vi "Teleop.vi"(10 "Match Info":T1={"Autonomous Elapsed Seconds"=0.0, "TeleOp Elapsed Seconds"=0.0, "Disabled Elapsed Seconds"=0.0, "Visited Autonomous"=FALSE, "Visited TeleOp"=FALSE, "Visited Disabled"=FALSE, "Autonomous Settings"={"Autonomous Style"=enum."Independent", "VI Refnum"=refnum}}, 11 "Call Context":T2) -> ()   [LabVIEW 2014]
doc: "This VI is called for each TeleOp packet received from the DS where the robot is not disabled. It is often used to read from the joysticks and update I/O or to update setpoints for timed control loops. It should complete and return within 20 milliseconds or it may miss DS packets."
uses:
  <vilib>/Rock Robotics/WPI/DriverStation/WPI_DriverStationDerivedRobotMode.ctl
  <vilib>/Rock Robotics/WPI/DriverStation/WPI_DriverStationMatch Info.ctl
  <vilib>/Rock Robotics/Network Tables/SD Read Boolean.vi
  <vilib>/Rock Robotics/Network Tables/SD Read Number.vi
  <vilib>/Rock Robotics/WPI/Joystick/WPI_JoystickGetSetRefNum.vi
  <vilib>/Rock Robotics/WPI/RobotDrive/WPI_RobotDriveGetSetRefNum.vi
  <vilib>/Rock Robotics/Network Tables/SD Write Numeric Array.vi
  <vilib>/Rock Robotics/Network Tables/SD Write Boolean Array.vi
panel:
  out "Right and Left Drive Motors Indicator":dbl[](array[numeric])
  out "Winch Cim 2 Indicator":dbl
  out "Winch Cim 1 Indicator":dbl
  out "Lower Limit Indicator":bool
  out "Back Ejector Limit Indicator":bool
  out "Left Drive Encoder Indicator":dbl
  out "Right Drive Encoder Indicator":dbl
  out "Front Ejector Limit Indicator":bool
  out "Claw Open Limit Indicator":bool
  out "Claw Closed Limit Indicator":bool
  out "Upper Limit Indicator":bool
  out "Buttons":bool[](array[boolean])
  out "Axes":dbl[](array[numeric])
  out "Sample Slider 0":dbl(slide) scale=0.0..5.0
  out "Sample Boolean 1":bool
  out "Sample Boolean 0":bool
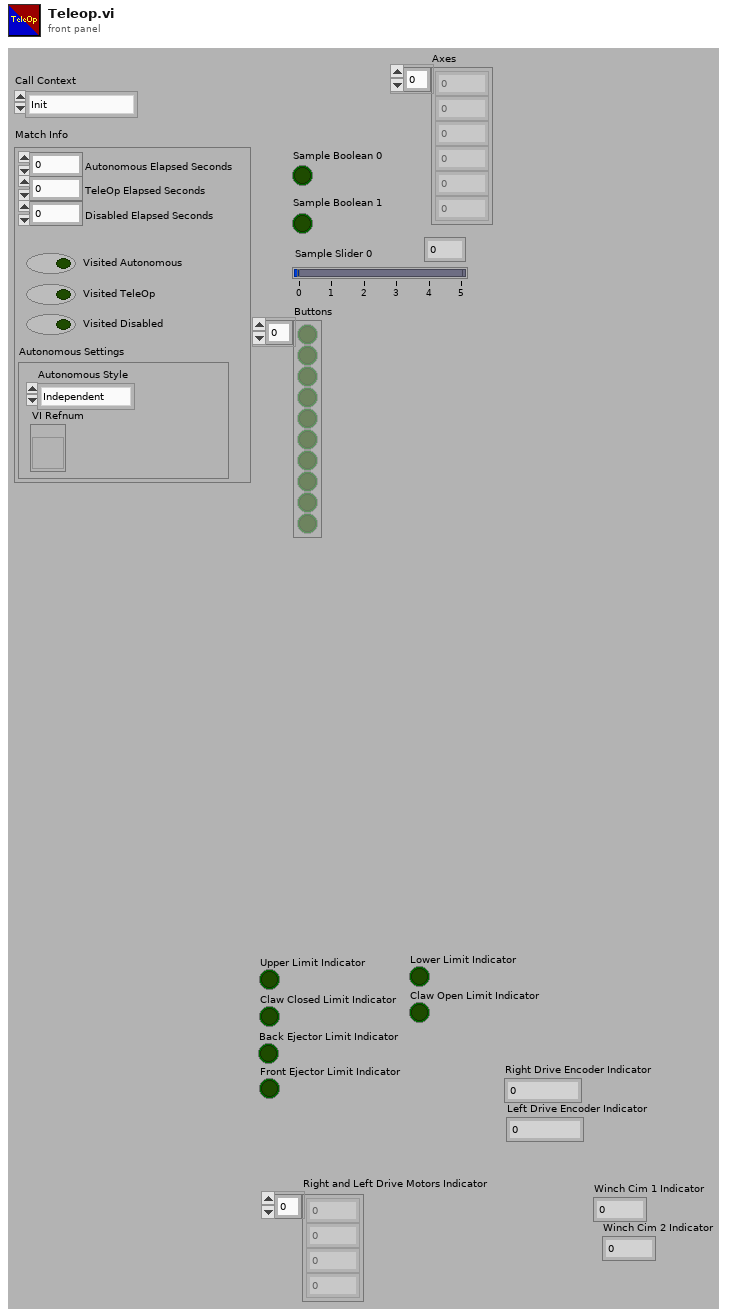
[diagram p1: front panel]
types:
  T1 = typedef "WPI_DriverStationMatch Info.ctl" = cluster{"Autonomous Elapsed Seconds":dbl, "TeleOp Elapsed Seconds":dbl, "Disabled Elapsed Seconds":dbl, "Visited Autonomous":bool, "Visited TeleOp":bool, "Visited Disabled":bool, "Autonomous Settings":cluster{"Autonomous Style":enum16{"Iterative", "Independent"}, "VI Refnum":refnum<vi>}}
  T2 = typedef "WPI_DriverStationDerivedRobotMode.ctl" = enum16{"Init", "Execute", "Stop"}
  T3 = typedef "WPI_RobotDriveDevRef.ctl" = cluster{"DevStatus":errorcluster, "Motors[]":T4[], "Square Inputs":bool, "Max Output":dbl}
  T4 = typedef "WPI_MotorControlDeviceRef.ctl" = cluster{"DeviceStatus":errorcluster, "Type":T5, "PWM":cluster{"Controller":T6, "PWM Channel":T7, "DeadBand":T8}, "CAN":cluster{"Device Number":u8, "Control Mode":T9, "Semaphore":T10, "Max Vout":dbl, "TalonSRX Control Mode":T11}, "Invert":bool, "TransformRef":T12, "InvTransformRef":T12}
  T5 = typedef "WPI_MotorControlType.ctl" = enum16{"PWM", "CAN", "CANTalonSRX"}
  T6 = typedef "FPGA_TypedefDigitalModule.ctl" = enum16{"Controller 1"}
  T7 = typedef "FPGA_DIOPWMChannel.ctl" = enum8{"PWM 0", "PWM 1", "PWM 2", "PWM 3", "PWM 4", "PWM 5", "PWM 6", "PWM 7", "PWM 8", "PWM 9", "PWM MXP 0", "PWM MXP 1", "PWM MXP 2", "PWM MXP 3", "PWM MXP 4", "PWM MXP 5", "PWM MXP 6", "PWM MXP 7", "PWM MXP 8", "PWM MXP 9", "Invalid"}
  T8 = typedef "WPI_PWMDeadband.ctl" = cluster{"Name":string, "maxPositivePwm":i32, "minPositivePwm":i32, "centerPwm":i32, "maxNegativePwm":i32, "minNegativePwm":i32, "angularRange":u16}
  T9 = typedef "WPI_CANJaguar_ControlMode.ctl" = enum8{"Percent VBus", "Current", "Speed", "Position", "Voltage"}
  T10 = typedef "Semaphore RefNum" = refnum<k1>
  T11 = typedef "WPI_CANTalonSRX_APIControlMode.ctl" = enum8{"Percent VBus", "Speed", "Position", "Slave", "Unchanged / Invalid"}
  T12 = typedef "WPI_PWMTransform_ConPane.ctl" = refnum<vi>
  T13 = typedef "WPI_JoystickDevRef.ctl" = cluster{"Device":T14}
  T14 = typedef "WPI_JoystickDeviceEnum.ctl" = enum16{"USB 0", "USB 1", "USB 2", "USB 3", "USB 4", "USB 5"}
  T15 = cluster{"Axes[0]":dbl, "Axes[1]":dbl, "Axes[2]":dbl, "Axes[3]":dbl, "Axes[4]":dbl, "Axes[5]":dbl, "Axes[6]":dbl, "Axes[7]":dbl, "Axes[8]":dbl}
  T16 = cluster{"Buttons[0]":bool, "Buttons[1]":bool, "Buttons[2]":bool, "Buttons[3]":bool, "Buttons[4]":bool, "Buttons[5]":bool, "Buttons[6]":bool, "Buttons[7]":bool, "Buttons[8]":bool}
  T17 = typedef "WPI_DigitalInputDevRef.ctl" = cluster{"DevStatus":errorcluster, "DIO Channel":T18, "Controller":T6}
  T18 = typedef "FPGA_DIOChannel.ctl" = enum8{"DIO 0", "DIO 1", "DIO 2", "DIO 3", "DIO 4", "DIO 5", "DIO 6", "DIO 7", "DIO 8", "DIO 9", "DIO MXP 0", "DIO MXP 1", "DIO MXP 2", "DIO MXP 3", "DIO MXP 4", "DIO MXP 5", "DIO MXP 6", "DIO MXP 7", "DIO MXP 8", "DIO MXP 9", "DIO MXP 10", "DIO MXP 11", "DIO MXP 12", "DIO MXP 13", "DIO MXP 14", "DIO MXP 15", "Invalid"}
  T19 = typedef "WPI_EncoderDevRef.ctl" = cluster{"DevStatus":errorcluster, "EncoderIndex":T20, "CounterIndex":T21, "DistancePerCount":dbl, "Decoding Type":T22}
  T20 = typedef "FPGA_EncoderIdx.ctl" = enum8{"Enc 0", "Enc 1", "Enc 2", "Enc 3", "Enc 4", "Enc 5", "Enc 6", "Enc 7", "Invalid"}
  T21 = typedef "FPGA_CounterCtrSystemIndex.ctl" = enum8{"Ctr 0", "Ctr 1", "Ctr 2", "Ctr 3", "Ctr 4", "Ctr 5", "Ctr 6", "Ctr 7", "Invalid"}
  T22 = typedef "WPI_EncoderType.ctl" = enum16{"1x", "2x", "4x"}
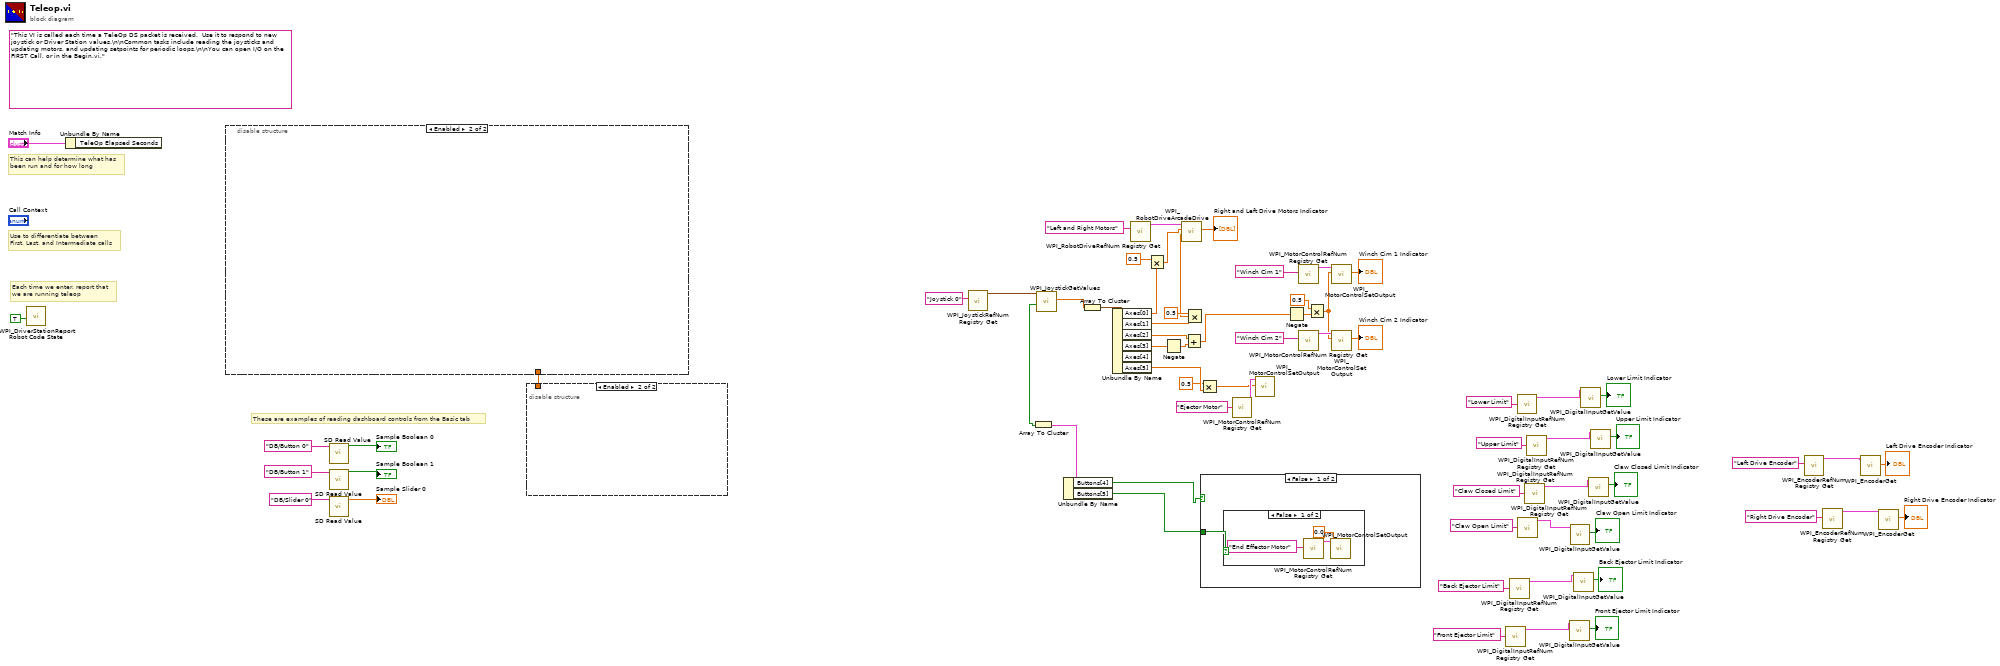
[diagram p0: block diagram]
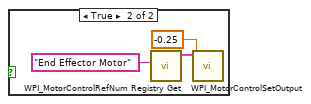
[diagram p2: hidden frame]
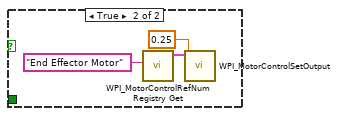
[diagram p3: hidden frame]
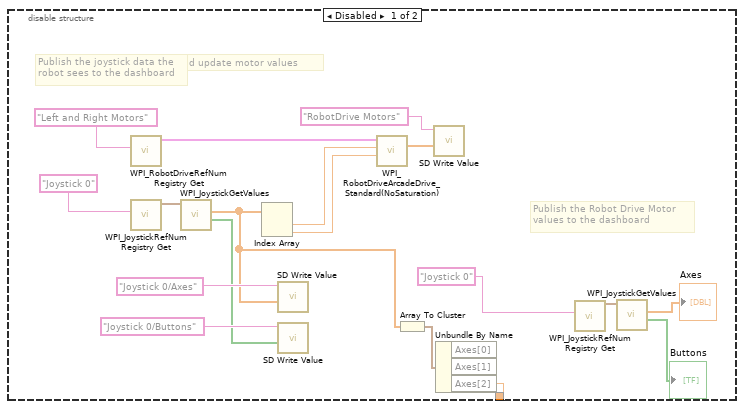
[diagram p4: hidden frame]
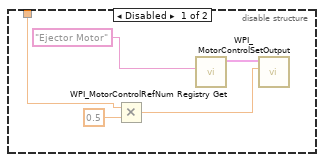
[diagram p5: hidden frame]
diagram:
  (unwired) "This VI is called each time a TeleOp DS packet is received.  Use it to respond to new joystick or Driver Station values.\n\nCommon tasks include reading the joysticks and updating motors, and updating setpoints for periodic loops.\n\nYou can open I/O on the FIRST Call, or in the Begin.vi."
  # "These are examples of reading dashboard controls from the Basic tab"
  # "Each time we enter, report that\nwe are running teleop"
  # "Use to differentiate between\nFirst, Last, and Intermediate calls"
  # "This can help determine what has\nbeen run and for how long"
  n1 = call <vilib>:"WPI_DriverStationReport Robot Code State.vi"("TeleOp"=TRUE ("Autonomous")) -> ()  [unwired: 10 in, 1 out]
  n2 = Unbundle By Name("Match Info") -> ()  [unwired: 1 out]
  n3 = disable-structure shown="Enabled" {
    disable-tunnel: [w69 _] -> w60
    frame Disabled {
      # "Publish the Robot Drive Motor\nvalues to the dashboard"
      # "Publish the joystick data the\nrobot sees to the dashboard"
      # "Read Joystick X and Y values and update motor values"
      n4 = call <vilib>:"WPI_RobotDriveRefNum Registry Get.vi"("refnum name"="Left and Right Motors") -> ("RobotDriveDevRef"=w85:T3)  [unwired: 1 in, 9 out]
      n5 = call <vilib>:"WPI_JoystickRefNum Registry Get.vi"("refnum name"="Joystick 0") -> ("JoystickDevRef"=w82:T13)  [unwired: 1 in, 9 out]
      n6 = call <vilib>:"WPI_JoystickGetValues.vi"("JoystickDevRef"=w82) -> ("Buttons"=w76:bool[], "Axes"=w71:dbl[])  [unwired: 6 in, 3 out]
      n7 = Index Array(array=w71) -> (element #1=w84:dbl, element #2=w80:dbl)  [unwired: 2 in]
      n8 = call-poly <vilib>:"SD Write Value.vi"("Numeric Array"=w71, "Name"="Joystick 0/Axes") -> ()  [unwired: 8 in, 2 out]
      n9 = call-poly <vilib>:"SD Write Value.vi"("Boolean Array"=w76, "Name"="Joystick 0/Buttons") -> ()  [unwired: 8 in, 2 out]
      n10 = call <vilib>:"WPI_RobotDriveArcadeDrive_Standard(NoSaturation).vi"("Y axis value"=w80, "X axis value"=w84, "RobotDriveDevRef"=w85) -> ("Motor Values"=w79:dbl[])  [unwired: 1 in, 7 out]
      n11 = Array To Cluster(array=w71) -> (cluster=w70:T15)
      n12 = call-poly <vilib>:"SD Write Value.vi"("Numeric Array"=w79, "Name"="RobotDrive Motors") -> ()  [unwired: 8 in, 2 out]
      n13 = Unbundle By Name(w70) -> ("Axes[2]"=w69:dbl)  [unwired: 2 out]
      n14 = call <vilib>:"WPI_JoystickRefNum Registry Get.vi"("refnum name"="Joystick 0") -> ("JoystickDevRef"=w74:T13)  [unwired: 9 in, 1 out]
      n15 = call <vilib>:"WPI_JoystickGetValues.vi"("JoystickDevRef"=w74) -> ("Buttons"=→"Buttons":bool[], "Axes"=→"Axes":dbl[])  [unwired: 6 in, 3 out]
    }
    frame Enabled {
    }
  }
  n16 = call-poly <vilib>:"SD Read Value.vi"("Name"="DB/Button 0" ("refnum name")) -> ("Boolean"=→"Sample Boolean 0":bool)  [unwired: 8 in, 2 out]
  n17 = call-poly <vilib>:"SD Read Value.vi"("Name"="DB/Button 1" ("refnum name")) -> ("Boolean"=→"Sample Boolean 1":bool)  [unwired: 8 in, 2 out]
  n18 = call-poly <vilib>:"SD Read Value.vi"("Name"="DB/Slider 0" ("refnum name")) -> ("Numeric"=→"Sample Slider 0":dbl)  [unwired: 8 in, 2 out]
  n19 = disable-structure shown="Enabled" {
    disable-tunnel: w60 -> [w88 _]
    frame Disabled {
      n20 = Multiply(x=w88, y=0.5) -> (x*y=w87:dbl)
      n21 = call <vilib>:"WPI_MotorControlRefNum Registry Get.vi"("refnum name"="Ejector Motor") -> ("MotorControlDevRef"=w90:T4)  [unwired: 9 in, 1 out]
      n22 = call <vilib>:"WPI_MotorControlSetOutput.vi"("Output"=w87, "MotorControlDevRef"=w90) -> ()  [unwired: 7 in, 3 out]
    }
    frame Enabled {
    }
  }
  n23 = call <vilib>:"WPI_JoystickRefNum Registry Get.vi"("refnum name"="Joystick 0") -> ("JoystickDevRef"=w37:T13)  [unwired: 9 in, 1 out]
  n24 = call <vilib>:"WPI_JoystickGetValues.vi"("JoystickDevRef"=w37) -> ("Buttons"=w33:bool[], "Axes"=w35:dbl[])  [unwired: 6 in, 3 out]
  n25 = Array To Cluster(array=w33) -> (cluster=w32:T16)
  n26 = Unbundle By Name(w32) -> ("Buttons[4]"=w5:bool, "Buttons[5]"=w4:bool)
  n27 = Array To Cluster(array=w35) -> (cluster=w34:T15)
  n28 = Unbundle By Name(w34) -> ("Axes[0]"=w7:dbl, "Axes[1]"=w11:dbl, "Axes[2]"=w20:dbl, "Axes[3]"=w21:dbl, "Axes[5]"=w2:dbl)  [unwired: 1 out]
  n29 = call <vilib>:"WPI_RobotDriveRefNum Registry Get.vi"("refnum name"="Left and Right Motors") -> ("RobotDriveDevRef"=w31:T3)  [unwired: 9 in, 1 out]
  n30 = Multiply(x=0.5, y=w7) -> (x*y=w6:dbl)
  n31 = Negate(x=w21) -> (-x=w19:dbl)
  n32 = Add(x=w20, y=w19) -> (x+y=w3:dbl)
  n33 = Multiply(x=0.5, y=w11) -> (x*y=w9:dbl)
  n34 = call-poly <vilib>:"WPI_RobotDriveArcadeDrive.vi"("Y axis value"=w9, "X axis value"=w6, "RobotDriveDevRef"=w31) -> ("Motor Values"=→"Right and Left Drive Motors Indicator":dbl[])  [unwired: 6 in, 2 out]
  n35 = Multiply(x=0.5, y=w2) -> (x*y=w12:dbl)
  n36 = case shown="False" w5 {
    tunnel: w4 -> [w92 _]
    frame False {
      n37 = case shown="False" w92 {
        frame False {
          n38 = call <vilib>:"WPI_MotorControlRefNum Registry Get.vi"("refnum name"="End Effector Motor" ("Name")) -> ("MotorControlDevRef"=w95:T4)  [unwired: 9 in, 1 out]
          n39 = call <vilib>:"WPI_MotorControlSetOutput.vi"("Output"=0.0, "MotorControlDevRef"=w95) -> ()  [unwired: 7 in, 3 out]
        }
        frame True {
          n40 = call <vilib>:"WPI_MotorControlRefNum Registry Get.vi"("refnum name"="End Effector Motor" ("Name")) -> ("MotorControlDevRef"=w98:T4)  [unwired: 9 in, 1 out]
          n41 = call <vilib>:"WPI_MotorControlSetOutput.vi"("Output"=-0.25, "MotorControlDevRef"=w98) -> ()  [unwired: 7 in, 3 out]
        }
      }
    }
    frame True {
      n42 = call <vilib>:"WPI_MotorControlRefNum Registry Get.vi"("refnum name"="End Effector Motor" ("Name")) -> ("MotorControlDevRef"=w101:T4)  [unwired: 9 in, 1 out]
      n43 = call <vilib>:"WPI_MotorControlSetOutput.vi"("Output"=0.25, "MotorControlDevRef"=w101) -> ()  [unwired: 7 in, 3 out]
    }
  }
  n44 = call <vilib>:"WPI_MotorControlRefNum Registry Get.vi"("refnum name"="Ejector Motor" ("Name")) -> ("MotorControlDevRef"=w55:T4)  [unwired: 9 in, 1 out]
  n45 = call <vilib>:"WPI_MotorControlSetOutput.vi"("Output"=w12, "MotorControlDevRef"=w55) -> ()  [unwired: 7 in, 3 out]
  n46 = Negate(x=w3) -> (-x=w15:dbl)
  n47 = call <vilib>:"WPI_MotorControlRefNum Registry Get.vi"("refnum name"="Winch Cim 1" ("Name")) -> ("MotorControlDevRef"=w59:T4)  [unwired: 9 in, 1 out]
  n48 = call <vilib>:"WPI_MotorControlRefNum Registry Get.vi"("refnum name"="Winch Cim 2" ("Name")) -> ("MotorControlDevRef"=w57:T4)  [unwired: 9 in, 1 out]
  n49 = Multiply(x=0.5, y=w15) -> (x*y=w13:dbl)
  n50 = call <vilib>:"WPI_MotorControlSetOutput.vi"("Output"=w13, "MotorControlDevRef"=w59) -> ("Motor Output"=→"Winch Cim 1 Indicator":dbl)  [unwired: 7 in, 2 out]
  n51 = call <vilib>:"WPI_MotorControlSetOutput.vi"("Output"=w13, "MotorControlDevRef"=w57) -> ("Motor Output"=→"Winch Cim 2 Indicator":dbl)  [unwired: 7 in, 2 out]
  n52 = call <vilib>:"WPI_DigitalInputRefNum Registry Get.vi"("refnum name"="Front Ejector Limit") -> ("DigitalInputDevRef"=w45:T17)  [unwired: 9 in, 1 out]
  n53 = call <vilib>:"WPI_DigitalInputRefNum Registry Get.vi"("refnum name"="Back Ejector Limit") -> ("DigitalInputDevRef"=w43:T17)  [unwired: 9 in, 1 out]
  n54 = call <vilib>:"WPI_DigitalInputRefNum Registry Get.vi"("refnum name"="Lower Limit") -> ("DigitalInputDevRef"=w49:T17)  [unwired: 9 in, 1 out]
  n55 = call <vilib>:"WPI_DigitalInputRefNum Registry Get.vi"("refnum name"="Claw Open Limit") -> ("DigitalInputDevRef"=w47:T17)  [unwired: 9 in, 1 out]
  n56 = call <vilib>:"WPI_DigitalInputRefNum Registry Get.vi"("refnum name"="Claw Closed Limit") -> ("DigitalInputDevRef"=w51:T17)  [unwired: 9 in, 1 out]
  n57 = call <vilib>:"WPI_DigitalInputRefNum Registry Get.vi"("refnum name"="Upper Limit") -> ("DigitalInputDevRef"=w53:T17)  [unwired: 9 in, 1 out]
  n58 = call <vilib>:"WPI_DigitalInputGetValue.vi"("DigitalInputDevRef"=w45) -> ("Value"=→"Front Ejector Limit Indicator":bool)  [unwired: 8 in, 2 out]
  n59 = call <vilib>:"WPI_DigitalInputGetValue.vi"("DigitalInputDevRef"=w47) -> ("Value"=→"Claw Open Limit Indicator":bool)  [unwired: 8 in, 2 out]
  n60 = call <vilib>:"WPI_DigitalInputGetValue.vi"("DigitalInputDevRef"=w43) -> ("Value"=→"Back Ejector Limit Indicator":bool)  [unwired: 8 in, 2 out]
  n61 = call <vilib>:"WPI_DigitalInputGetValue.vi"("DigitalInputDevRef"=w49) -> ("Value"=→"Lower Limit Indicator":bool)  [unwired: 8 in, 2 out]
  n62 = call <vilib>:"WPI_DigitalInputGetValue.vi"("DigitalInputDevRef"=w51) -> ("Value"=→"Claw Closed Limit Indicator":bool)  [unwired: 8 in, 2 out]
  n63 = call <vilib>:"WPI_DigitalInputGetValue.vi"("DigitalInputDevRef"=w53) -> ("Value"=→"Upper Limit Indicator":bool)  [unwired: 8 in, 2 out]
  n64 = call <vilib>:"WPI_EncoderRefNum Registry Get.vi"("refnum name"="Left Drive Encoder") -> ("EncoderDevRef"=w41:T19)  [unwired: 9 in, 1 out]
  n65 = call <vilib>:"WPI_EncoderRefNum Registry Get.vi"("refnum name"="Right Drive Encoder") -> ("EncoderDevRef"=w39:T19)  [unwired: 9 in, 1 out]
  n66 = call <vilib>:"WPI_EncoderGet.vi"("EncoderDevRef"=w41) -> ("Distance"=→"Left Drive Encoder Indicator":dbl)  [unwired: 5 in, 5 out]
  n67 = call <vilib>:"WPI_EncoderGet.vi"("EncoderDevRef"=w39) -> ("Distance"=→"Right Drive Encoder Indicator":dbl)  [unwired: 5 in, 5 out]
